vi "RGB Depth To Grayscale Depth.vi"(1 "Image Dest.":T1, 2 "RGB Depth Image":T1) -> (0 "Grayscale Depth Image":T1)   [LabVIEW 2018]
uses:
  <vilib>/vision/Image Controls.llb/IMAQ Image.ctl
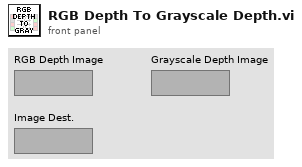
[diagram p1: front panel]
types:
  T1 = typedef "IMAQ Image.ctl" = refnum<image>
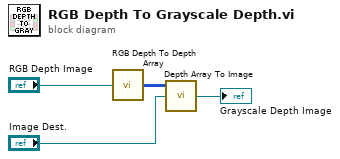
[diagram p0: block diagram]
diagram:
  n1 = call "RGB Depth To Depth Array.vi"("RGB Image"="RGB Depth Image") -> ("Depth Array"=w3:u16[][])
  n2 = call "Depth Array To Image.vi"("Image Dest."="Image Dest.", "Depth Array"=w3) -> ("Image out"=→"Grayscale Depth Image":T1)  [unwired: 3 in]
